vi "play_AFM_PI_trajTrack.vi"() -> ()   [LabVIEW 2017]
uses:
  controls/controlParams_tracktraj.ctl
  <vilib>/userdefined/High Color/nirio_resource_hc.ctl
  <vilib>/Utility/file.llb/Read From Spreadsheet File (DBL).vi
  <vilib>/FPGAPlugInAG/cRIO-9082/niLvFpga_Open_cRIO-9082.vi
  <vilib>/rvi/interface/common/dynamic/niFpgaDynamicAddResources.vi
  <vilib>/FPGAPlugInAG/Dynamic/niLvFpga_Reset_Dynamic.vi
  <vilib>/rvi/interface/common/niFpgaWaitOnOcc.vi
  <vilib>/Utility/error.llb/Error Cluster From Error Code.vi
  <vilib>/rvi/errors/niLvFpgaAdjustHostInterfaceError.vi
  <vilib>/FPGAPlugInAG/Dynamic/niLvFpga_Run_Dynamic.vi
  <vilib>/Utility/file.llb/Write To Spreadsheet File (DBL).vi
  <vilib>/FPGAPlugInAG/Dynamic/niLvFpga_Close_Dynamic.vi
  <vilib>/rvi/interface/nirviOpenFPGA/nirviOpenFPGA.xnode
  FPGA Bitfiles/XYpeizocontrol_FPGATargetSPARTA_AFMPIcontroltraj_qMjg6HTFwTs.lvbitx
  <vilib>/rvi/interface/nirviMethod/nirviMethod.xnode
  <vilib>/rvi/interface/nirviReadWriteControl/nirviReadWriteControl.xnode
  <vilib>/rvi/interface/nirviCloseFPGA/nirviCloseFPGA.xnode
  <vilib>/FPGAPlugInAG/Dynamic/niLvFpga_ConfigureFifo_Dynamic.vi
  <vilib>/rvi/errors/niLvFpgaMergeErrorWithErrorCode.vi
  <vilib>/rvi/interface/Simulation/niFpgaSimulationCallBeginRW.vi
  <vilib>/FPGAPlugInAG/Dynamic/niLvFpga_ReadFifo_Dynamic.vi
  NiFpgaLv.dll
  <vilib>/FPGAPlugInAG/Dynamic/niLvFpga_WriteFifo_Dynamic.vi
panel:
  in  "Ki":dbl=0.125346917944 format="%#_13g"
  out "Actual Depth":u32
  out "YK TO":bool
  out "UK TO":bool
  out "yk":sgl
  out "loop ticks benchmark":sgl
  in  "Cluster":T1={"umax"=3.0, "y_ref(k)"=0.0, "Ki"=0.0, "y(k) (from plant)"=0.0, "ND"=0, "NS"=0, "u_Kx_ref(k)"=0.0} {"u_Kx_ref(k)" format="%#_13g"; "Ki" format="%#_13g"; "y_ref(k)" format="%#_13g"; "umax" format="%#_13g"}
  out "Unstable Traj":bool
  out "Control Loop Done":bool
  out "Elements Remaining":u32
  in  "reference traj path":path=path "Z:/mpc-journal/step-exps/ref_traj_track.csv"
  in  "outputData BOTH":path=path "Z:/mpc-journal/step-exps/exp01outputBOTH.csv"
  out "x+1":i32
  in  "SettleTicks":i32=10
  in  "Stop":bool=TRUE
  out "y iter":i32
  out "u iter":i32
  out "size(s) 5":i32
  out "size(s)":i32
  in  "Iters":i32=25
  in  "Cont Run (F)":bool=TRUE
  in  "ymax":dbl=4.0 format="%#_13g"
  in  "umax":dbl=1.0 format="%#_13g"
  in  "TsTicks":i32=1600
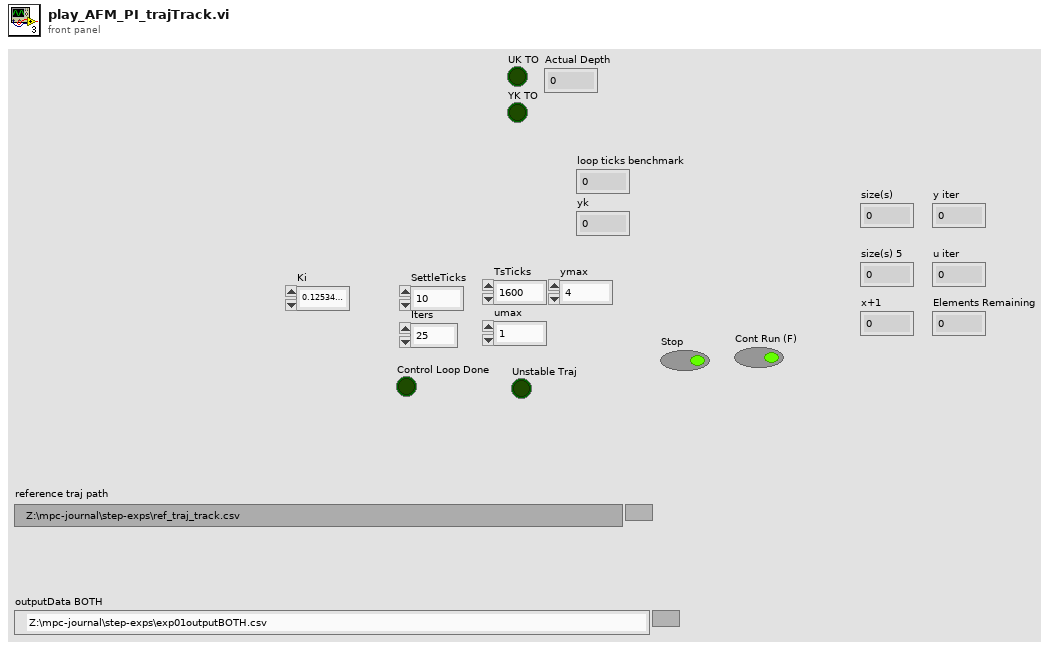
[diagram p1: front panel]
types:
  T1 = typedef "controlParams_tracktraj.ctl" = cluster{"umax":sgl, "y_ref(k)":sgl, "Ki":sgl, "y(k) (from plant)":sgl, "ND":i16, "NS":i16, "u_Kx_ref(k)":sgl}
  T2 = typedef "nirio_resource_hc.ctl" = tag
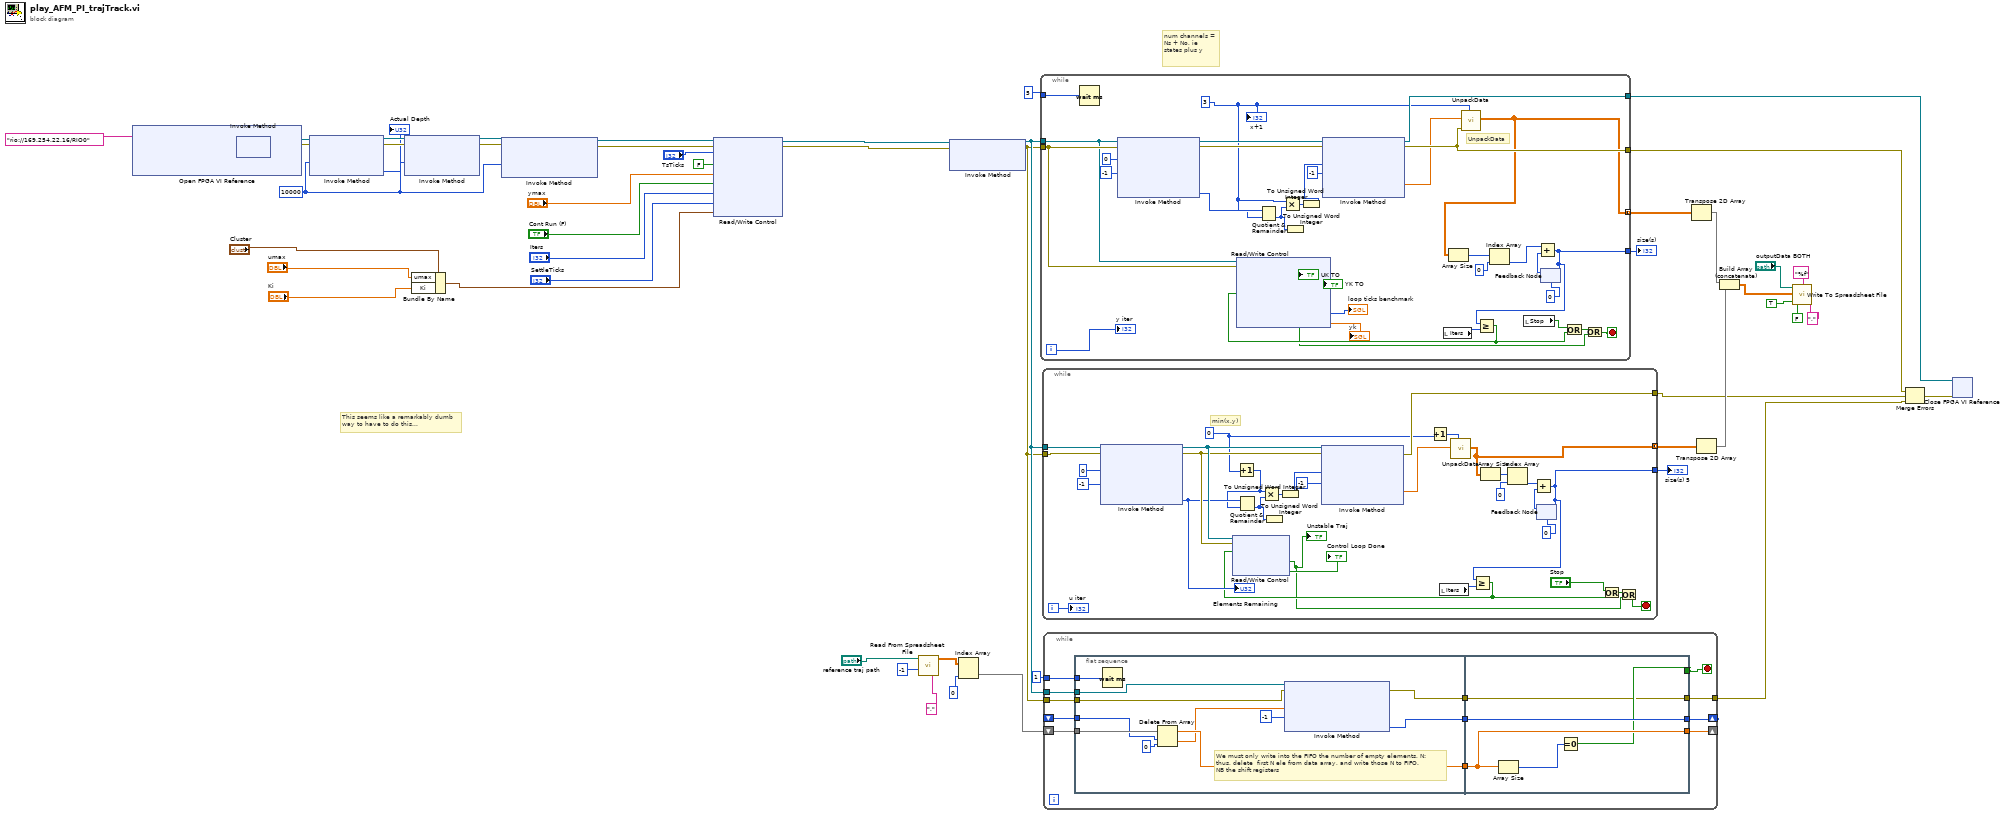
[diagram p0: block diagram]
diagram:
  w33 = 10000
  # "This seems like a remarkably dumb\nway to have to do this..."
  # "num channels = Ns + No, ie states plus y"
  n1 = xnode "Open FPGA VI Reference"("resource name"=T2 "rio://169.254.22.16/RIO0") -> ("FPGA VI Reference Out"=w31:refnum<k20>, "error out"=w30:errorcluster)  [unwired: 1 in]
  n2 = xnode "Invoke Method"("FPGA VI Reference In"=w31, "error in"=w30) -> ("FPGA VI Reference Out"=w40:refnum<k20>, "error out"=w39:errorcluster)
  n3 = xnode "Invoke Method"("FPGA VI Reference In"=w40, "error in"=w39, "Requested Depth"=w33) -> ("FPGA VI Reference Out"=w52:refnum<k20>, "error out"=w51:errorcluster, "Actual Depth"=→"Actual Depth":u32)
  n4 = xnode "Invoke Method"("FPGA VI Reference In"=w52, "error in"=w51, "Requested Depth"=w33) -> ("FPGA VI Reference Out"=w37:refnum<k20>, "error out"=w36:errorcluster)  [unwired: 1 out]
  n5 = Bundle By Name(cluster="Cluster", "umax"="umax", "Ki"="Ki") -> (w8:T1)
  n6 = xnode "Invoke Method"("FPGA VI Reference In"=w37, "error in"=w36, "Requested Depth"=w33) -> ("FPGA VI Reference Out"=w35:refnum<k20>, "error out"=w34:errorcluster)  [unwired: 1 out]
  n7 = xnode "Read/Write Control"("FPGA VI Reference In"=w35, "error in"=w34, "TsTicks"="TsTicks", "Abort"=FALSE, "ymax"="ymax", "False  = cont run"="Cont Run (F)", "iters"="Iters", "Settle Ticks"="SettleTicks", "Cluster"=w8) -> ("FPGA VI Reference Out"=w2:refnum<k20>, "error out"=w3:errorcluster)
  n8 = call-poly <vilib>:"Read From Spreadsheet File.vi"("delimiter (\\t)"=",", "number of rows (all:-1)"=-1, "file path (dialog if empty)"="reference traj path") -> ("all rows"=w15:dbl[][])  [unwired: 4 in, 4 out]
  n9 = xnode "Invoke Method"("FPGA VI Reference In"=w2, "error in"=w3) -> ("FPGA VI Reference Out"=w7:refnum<k20>, "error out"=w6:errorcluster)  [unwired: 1 in]
  n10 = Index Array(array=w15, index (col)=0 ("dimension size")) -> (element=w13:dbl[])  [unwired: 1 in]
  n11 = while {
    tunnel: 5 -> [w86]
    tunnel: w7 -> [w66]
    tunnel: w6 -> [w67]
    tunnel: [w78] -> w12
    tunnel: [w77] -> w44
    tunnel: [w65] -> w43 mode=concatenating
    tunnel: [w63] -> w41
    i -> [w64]
    stop <- w58 stop-if-true
    w53 = 3
    # "UnpackData"
    n12 = Wait (ms)(milliseconds to wait=w86) -> ()  [unwired: 1 out]
    n13 = xnode "Invoke Method"("FPGA VI Reference In"=w66, "error in"=w67, "Number of Elements"=0 ("Timeout (ms)"), "Timeout (ms)"=-1) -> ("FPGA VI Reference Out"=w82:refnum<k20>, "error out"=w83:errorcluster, "Elements Remaining"=w73:u32)  [unwired: 1 out]
    n14 = Quotient & Remainder(x=w73, y=w53) -> (floor(x/y)=w75:u32)  [unwired: 1 out]
    n15 = Multiply(x=w53, y=w75) -> (x*y=w80:u32)
    n16 = To Unsigned Word Integer(number=w75) -> ()  [unwired: 1 out]
    n17 = To Unsigned Word Integer(number=w80) -> (unsigned 16bit integer=w76:u16)
    n18 = xnode "Invoke Method"("FPGA VI Reference In"=w82, "error in"=w83, "Number of Elements"=w76, "Timeout (ms)"=-1) -> ("FPGA VI Reference Out"=w77:refnum<k20>, "error out"=w78:errorcluster, "Data"=w72:sgl[])  [unwired: 1 out]
    n19 = local read "Iters"() -> (w74:i32)
    n20 = call "UnpackData.vi"("NumChannels"=w53, "error In"=w78, "1D Data In"=w72) -> ("2D Data Out"=w65:dbl[][])  [unwired: 7 in, 1 out]
    n21 = Array Size(array=w65) -> (size(s)=w71:i32[])
    n22 = Index Array(array=w71, index=0) -> (element=w69:i32)
    n23 = local read "Stop"() -> (w61:bool)
    n24 = feedback #1(0) -> (w70:i32)
    n25 = Add(x=w69, y=w70) -> (x+y=w63:i32)
    n26 = Greater Or Equal?(x=w63, y=w74) -> (x >= y?=w62:bool)
    n27 = xnode "Read/Write Control"("FPGA VI Reference In"=w66, "error in"=w67, "Abort"=w62) -> ("UK TO"=→"UK TO":bool, "YK TO"=→"YK TO":bool, "Unstable Traj"=w59:bool, "Loop Ticks (benchmark)"=→"loop ticks benchmark":i16, "yk"=→"yk":sgl)  [unwired: 2 out]
    n28 = feedback-in #1(w63) -> ()
    n29 = Or(x=w61, y=w62) -> (x .or. y?=w60:bool)
    n30 = Or(x=w60, y=w59) -> (x .or. y?=w58:bool)
    "y iter" <- w64
    "x+1" <- w53
  }
  "size(s)" <- w41
  n31 = while {
    tunnel: [w96] -> w32 mode=concatenating
    tunnel: w7 -> [w104]
    tunnel: w6 -> [w103]
    tunnel: [w101] -> w42
    tunnel: [w92] -> w10
    i -> [w102]
    stop <- w91 stop-if-true
    w87 = i16 0 ("x")
    # "min(x,y)"
    n32 = xnode "Invoke Method"("FPGA VI Reference In"=w104, "error in"=w103, "Number of Elements"=0 ("Timeout (ms)"), "Timeout (ms)"=-1) -> ("FPGA VI Reference Out"=w112:refnum<k20>, "error out"=w111:errorcluster, "Elements Remaining"=w108:u32)  [unwired: 1 out]
    "Elements Remaining" <- w108
    n33 = Increment(x=w87) -> (x+1=w106:i16)
    n34 = Quotient & Remainder(x=w108, y=w106) -> (floor(x/y)=w109:u32)  [unwired: 1 out]
    n35 = Multiply(x=w106, y=w109) -> (x*y=w110:u32)
    n36 = To Unsigned Word Integer(number=w109) -> ()  [unwired: 1 out]
    n37 = To Unsigned Word Integer(number=w110) -> (unsigned 16bit integer=w107:u16)
    n38 = xnode "Invoke Method"("FPGA VI Reference In"=w112, "error in"=w111, "Number of Elements"=w107, "Timeout (ms)"=-1) -> ("error out"=w92:errorcluster, "Data"=w98:sgl[])  [unwired: 2 out]
    n39 = Increment(x=w87) -> (x+1=w95:i16)
    n40 = local read "Iters"() -> (w113:i32)
    n41 = call "UnpackData.vi"("NumChannels"=w95, "1D Data In"=w98) -> ("2D Data Out"=w96:dbl[][])  [unwired: 8 in, 1 out]
    n42 = Array Size(array=w96) -> (size(s)=w93:i32[])
    n43 = Index Array(array=w93, index=0) -> (element=w97:i32)
    n44 = feedback #2(0) -> (w105:i32)
    n45 = Add(x=w97, y=w105) -> (x+y=w101:i32)
    n46 = Greater Or Equal?(x=w101, y=w113) -> (x >= y?=w100:bool)
    n47 = xnode "Read/Write Control"("FPGA VI Reference In"=w112, "error in"=w111, "Abort"=w100) -> ("Unstable Traj"=w88:bool, "Loop Done"=→"Control Loop Done":bool)  [unwired: 2 out]
    "Unstable Traj" <- w88
    n48 = feedback-in #2(w101) -> ()
    n49 = Or(x="Stop", y=w100) -> (x .or. y?=w90:bool)
    n50 = Or(x=w90, y=w88) -> (x .or. y?=w91:bool)
    "u iter" <- w102
  }
  "size(s) 5" <- w42
  n51 = while {
    tunnel: [w127] -> w9
    tunnel: 1 -> [w129]
    shift-right: [w122] -> _
    shift-left: _ -> [w126]
    shift-right: [w120] -> _
    shift-left: w13 -> [w128]
    tunnel: w7 -> [w119]
    tunnel: w6 -> [w118]
    stop <- w123 stop-if-true
    n52 = flat-sequence {
      tunnel: w129 -> [w140]
      tunnel: w128 -> [w135]
      tunnel: w126 -> [w131]
      tunnel: [w138] -> w125
      tunnel: [w136] -> w124
      tunnel: [w137] -> w121
      tunnel: w119 -> [w133]
      tunnel: w118 -> [w132]
      tunnel: [w145] -> w122
      tunnel: [w141] -> w127
      tunnel: w125 -> [w141]
      tunnel: w124 -> [w145]
      tunnel: [w142] -> w123
      tunnel: w121 -> [w143]
      tunnel: [w143] -> w120
      frame #0 {
        # "We must only write into the FIFO the number of empty elements, N:\nthus, delete  first N ele from data array, and write those N to FIFO.\nNB the shift registers"
        n53 = Wait (ms)(milliseconds to wait=w140) -> ()  [unwired: 1 out]
        n54 = Delete From Array(array=w135, length=w131, index=0) -> (deleted portion=w134:dbl[], array with subset deleted=w137:dbl[])
        n55 = xnode "Invoke Method"("FPGA VI Reference In"=w133, "error in"=w132, "Data"=w134, "Timeout (ms)"=-1) -> ("error out"=w138:errorcluster, "Empty Elements Remaining"=w136:u32)  [unwired: 1 out]
      }
      frame #1 {
        n56 = Array Size(array=w143) -> (size(s)=w144:i32)
        n57 = Equal To 0?(x=w144) -> (x = 0?=w142:bool)
      }
    }
  }
  n58 = Transpose 2D Array(2D array=w43) -> (transposed array=w27:dbl[][])
  n59 = Transpose 2D Array(2D array=w32) -> (transposed array=w26:dbl[][])
  n60 = Build Array (concatenate)(w27, w26) -> (w20:dbl[][])
  n61 = call-poly <vilib>:"Write To Spreadsheet File.vi"("delimiter (\\t)"=",", "transpose? (no:F)"=TRUE, "format (%.3f)"="%f", "append to file? (new file:F)"=FALSE, "2D data"=w20, "file path (dialog if empty)"="outputData BOTH") -> ()  [unwired: 2 in, 1 out]
  n62 = Merge Errors(w12, w10, w9) -> (w11:errorcluster)
  n63 = xnode "Close FPGA VI Reference"("FPGA VI Reference In"=w44, "error in"=w11) -> ()  [unwired: 1 out]
